vi "MSScript_SubVI_EncolourExprSections.vi"(7 "TextProperties":T1={"Colour"=8404992, "Italic"=FALSE, "Bold"=TRUE}, 9 "Expression Sections":cluster{"Str":string, "Start":i32}[](array[cluster]), 10 "CMNT":cluster{"Start":u32, "End":u32}[](array[cluster]), 11 "String in":refnum<vi>) -> (0 "error out":errorcluster)   [LabVIEW 2018, in "MSScript.lvclass"]
uses:
  MSScript.lvclass
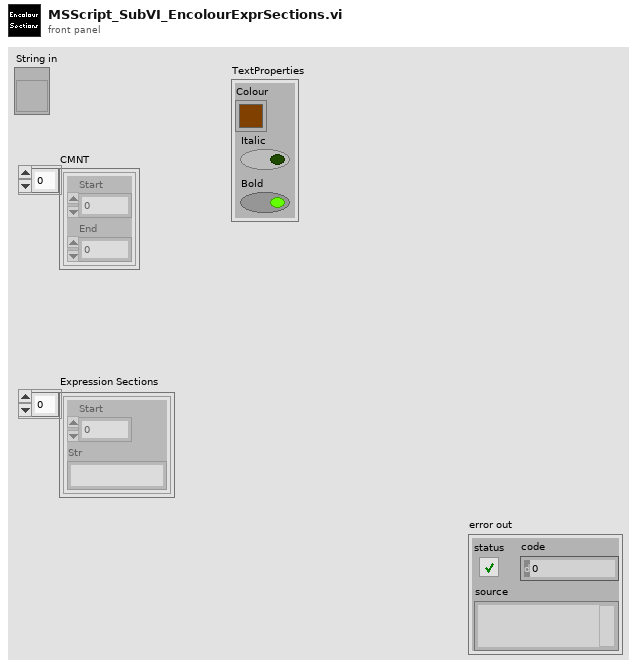
[diagram p1: front panel]
types:
  T1 = cluster{"Colour":u32, "Italic":bool, "Bold":bool}
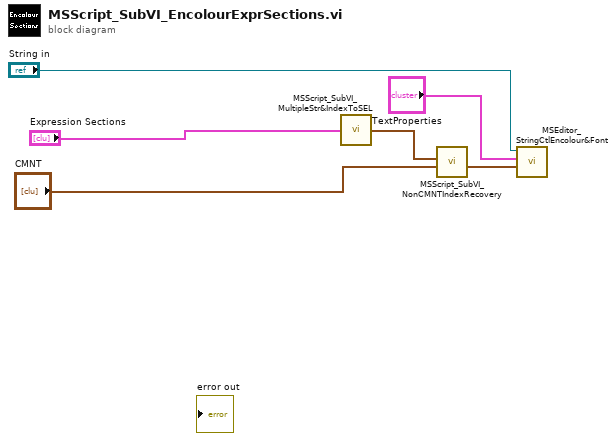
[diagram p0: block diagram]
diagram:
  n1 = call "MSScript_SubVI_MultipleStr&IndexToSEL.vi"("Expression Sections"="Expression Sections") -> ("SEL"=w2:cluster{"Start":u32, "End":u32}[])
  n2 = call "MSScript_SubVI_NonCMNTIndexRecovery.vi"("SEL of CMNT"="CMNT", "NonCMNT.SEL"=w2) -> ("RecoverySEL"=w4:cluster{"Start":u32, "End":u32}[])  [unwired: 5 in]
  n3 = call "MSEditor_StringCtlEncolour&Font.vi"("SELs"=w4, "TextProperties"="TextProperties", "String ctl ref"="String in") -> ()  [unwired: 7 in, 2 out]
